vi "OCV Host Client.vi"() -> ()   [LabVIEW 2019]
uses:
  OCVResults.ctl
  <vilib>/NI/STM/TCP/Read Meta Data (TCP Ref).vi
  <vilib>/NI/STM/TCP/Get Connection Reference (TCP).vi
  <vilib>/NI/STM/TCP/Read Meta Data (TCP Clst).vi
  <vilib>/NI/STM/TCP/Write Message (TCP).vi
  <vilib>/NI/STM/TCP/Read Message (TCP).vi
  <vilib>/NI/STM/NI STM.lvlib
panel:
  out "Results":T1={"V ch0 Array"=[-3.6706721797527737e-06, -3.7498129566879645e-06, -4.506527481324882e-06, -3.950514239764907e-06, -3.163693240167565e-06, -4.344248671038362e-06, -4.095274961024307e-06, -3.5751580182405744e-06, -3.679018613642735e-06, -4.241224075624106e-06, -3.987139173161142e-06, -4.095162898018893e-06, -3.847206102337771e-06, -3.5638421272775453e-06, -4.562072176859353e-06, -4.7605988032426154e-06, -4.427579247767526e-06, -3.852601385134958e-06, -4.1020189664170556e-06, -4.3281080989855496e-06, -5.440516492777152e-06, -3.984546752057509e-06, -5.212236089778075e-06, -5.036428159001794e-06, -5.147592315385633e-06, -5.639821151819425e-06, -5.515877149224325e-06, -4.719119249712352e-06, -4.963946714892732e-06, -5.484948605605908e-06, -4.699117481856034e-06, -4.371411013381793e-06], "V ch1 Array"=[3.16348946577608e-07, -4.6006644164974094e-08, 1.3969711256247924e-07, 5.504038021469118e-07, 6.043373546159048e-07, 8.588910763946214e-07, 3.873000478455866e-07, -9.425550832049107e-08, 5.478098926620833e-07, -1.5101867437911976e-08, 5.338250456123853e-07, 2.1443809689103476e-07, 4.7544765511864677e-07, 2.3162631910812704e-07, 8.243432281255722e-07, 4.471382249715257e-08, 5.99790680569682e-08, -2.2315078204485062e-07, 2.9341057780098417e-07, 5.004289692054384e-07, -7.392261536330597e-07, -5.620196062138411e-07, -3.660452758084688e-07, -9.194345360493777e-07, -9.111679257871997e-07, -7.512468979028726e-07, -1.0558354724851492e-06, -7.932704939374199e-07, -5.322755445721049e-07, -1.1027151194362871e-06, -8.832653614145757e-07, -1.2875743851160654e-08], "V ch2 Array"=[9.302674524081596e-06, 9.024588901172551e-06, 9.175881665259862e-06, 9.276460385887776e-06, 8.94756426004191e-06, 9.124853023363049e-06, 8.424398713182681e-06, 8.62613322878038e-06, 8.99729374546172e-06, 9.302350488450816e-06, 9.314432037131127e-06, 9.207132923863602e-06, 8.920051579064495e-06, 8.702882444652302e-06, 9.103302590152476e-06, 8.938969157386832e-06, 8.921195968554336e-06, 8.792009492927474e-06, 9.494545679269322e-06, 9.110247967355348e-06, 8.668435221623828e-06, 7.95156633600334e-06, 8.401197094566e-06, 8.499396743148332e-06, 8.067369388963132e-06, 8.816372879417737e-06, 7.610167561411513e-06, 7.594234882129245e-06, 8.485125121852154e-06, 8.105819415375889e-06, 8.729915422429432e-06, 7.897303713033343e-06], "V ch3 Array"=[7.69393857109199e-06, 8.057167587189197e-06, 7.1228622148927485e-06, 7.424852427233159e-06, 6.8217649437894305e-06, 7.201445944926346e-06, 7.710957721782108e-06, 7.736723821001707e-06, 7.68957282130428e-06, 7.319043173912174e-06, 7.476899876041569e-06, 7.1550863314873234e-06, 7.295375552383249e-06, 7.1219749115015865e-06, 7.996068874298418e-06, 7.215675170715944e-06, 7.2928039847892635e-06, 7.091536693290006e-06, 7.2765313907074405e-06, 7.659634434212023e-06, 7.289115911683562e-06, 6.62300445032373e-06, 6.310563673677977e-06, 6.475814441935722e-06, 6.9014245158358485e-06, 6.608592632669611e-06, 6.07353098569707e-06, 6.0353281126732675e-06, 6.4467487474758576e-06, 6.896290120465679e-06, 7.301165398420061e-06, 6.570120591901739e-06], "V ch4 Array"=[], "Elapsed Time (ms)"=5101, "DMM Fault Array"=[FALSE, FALSE, FALSE, FALSE, FALSE, FALSE, FALSE, FALSE, FALSE, FALSE, FALSE, FALSE, FALSE, FALSE, FALSE, FALSE, FALSE, FALSE, FALSE, FALSE, FALSE, FALSE, FALSE, FALSE, FALSE, FALSE, FALSE, FALSE, FALSE, FALSE, FALSE, FALSE, FALSE, FALSE, FALSE, FALSE, FALSE, FALSE, FALSE, FALSE, FALSE, FALSE, FALSE, FALSE, FALSE, FALSE, FALSE, FALSE, FALSE, FALSE, FALSE, FALSE, FALSE, FALSE, FALSE, FALSE, FALSE, FALSE, FALSE, FALSE, FALSE, FALSE, FALSE, FALSE, FALSE, FALSE, FALSE, FALSE, FALSE, FALSE, FALSE, FALSE, FALSE, FALSE, FALSE, FALSE, FALSE, FALSE, FALSE, FALSE, FALSE, FALSE, FALSE, FALSE, FALSE, FALSE, FALSE, FALSE, FALSE, FALSE, FALSE, FALSE, FALSE, FALSE, FALSE, FALSE, FALSE, FALSE, FALSE, FALSE, FALSE, FALSE, FALSE, FALSE, FALSE, FALSE, FALSE, FALSE, FALSE, FALSE, FALSE, FALSE, FALSE, FALSE, FALSE, FALSE, FALSE, FALSE, FALSE, FALSE, FALSE, FALSE, FALSE, FALSE, FALSE, FALSE, FALSE, FALSE]}
  out "Waveform Graph ch3":dbl[](graph)=[7.69393857109199e-06, 8.057167587189197e-06, 7.1228622148927485e-06, 7.424852427233159e-06, 6.8217649437894305e-06, 7.201445944926346e-06, 7.710957721782108e-06, 7.736723821001707e-06, 7.68957282130428e-06, 7.319043173912174e-06, 7.476899876041569e-06, 7.1550863314873234e-06, 7.295375552383249e-06, 7.1219749115015865e-06, 7.996068874298418e-06, 7.215675170715944e-06, 7.2928039847892635e-06, 7.091536693290006e-06, 7.2765313907074405e-06, 7.659634434212023e-06, 7.289115911683562e-06, 6.62300445032373e-06, 6.310563673677977e-06, 6.475814441935722e-06, 6.9014245158358485e-06, 6.608592632669611e-06, 6.07353098569707e-06, 6.0353281126732675e-06, 6.4467487474758576e-06, 6.896290120465679e-06, 7.301165398420061e-06, 6.570120591901739e-06]
  out "Waveform Graph ch2":dbl[](graph)=[9.302674524081596e-06, 9.024588901172551e-06, 9.175881665259862e-06, 9.276460385887776e-06, 8.94756426004191e-06, 9.124853023363049e-06, 8.424398713182681e-06, 8.62613322878038e-06, 8.99729374546172e-06, 9.302350488450816e-06, 9.314432037131127e-06, 9.207132923863602e-06, 8.920051579064495e-06, 8.702882444652302e-06, 9.103302590152476e-06, 8.938969157386832e-06, 8.921195968554336e-06, 8.792009492927474e-06, 9.494545679269322e-06, 9.110247967355348e-06, 8.668435221623828e-06, 7.95156633600334e-06, 8.401197094566e-06, 8.499396743148332e-06, 8.067369388963132e-06, 8.816372879417737e-06, 7.610167561411513e-06, 7.594234882129245e-06, 8.485125121852154e-06, 8.105819415375889e-06, 8.729915422429432e-06, 7.897303713033343e-06]
  out "Waveform Graph ch1":dbl[](graph)=[3.16348946577608e-07, -4.6006644164974094e-08, 1.3969711256247924e-07, 5.504038021469118e-07, 6.043373546159048e-07, 8.588910763946214e-07, 3.873000478455866e-07, -9.425550832049107e-08, 5.478098926620833e-07, -1.5101867437911976e-08, 5.338250456123853e-07, 2.1443809689103476e-07, 4.7544765511864677e-07, 2.3162631910812704e-07, 8.243432281255722e-07, 4.471382249715257e-08, 5.99790680569682e-08, -2.2315078204485062e-07, 2.9341057780098417e-07, 5.004289692054384e-07, -7.392261536330597e-07, -5.620196062138411e-07, -3.660452758084688e-07, -9.194345360493777e-07, -9.111679257871997e-07, -7.512468979028726e-07, -1.0558354724851492e-06, -7.932704939374199e-07, -5.322755445721049e-07, -1.1027151194362871e-06, -8.832653614145757e-07, -1.2875743851160654e-08]
  out "Scanning":bool
  out "Waveform Graph ch0":dbl[](graph)=[-3.6706721797527737e-06, -3.7498129566879645e-06, -4.506527481324882e-06, -3.950514239764907e-06, -3.163693240167565e-06, -4.344248671038362e-06, -4.095274961024307e-06, -3.5751580182405744e-06, -3.679018613642735e-06, -4.241224075624106e-06, -3.987139173161142e-06, -4.095162898018893e-06, -3.847206102337771e-06, -3.5638421272775453e-06, -4.562072176859353e-06, -4.7605988032426154e-06, -4.427579247767526e-06, -3.852601385134958e-06, -4.1020189664170556e-06, -4.3281080989855496e-06, -5.440516492777152e-06, -3.984546752057509e-06, -5.212236089778075e-06, -5.036428159001794e-06, -5.147592315385633e-06, -5.639821151819425e-06, -5.515877149224325e-06, -4.719119249712352e-06, -4.963946714892732e-06, -5.484948605605908e-06, -4.699117481856034e-06, -4.371411013381793e-06]
  in  "Command":string(combo)="Stop Client"
  out "Error Out":errorcluster={"status"=FALSE, "code"=66, "source"="TCP Read in NI STM.lvlib:Read Message (TCP).vi:6180001->OCV Host Client.vi"}
  in  "Send_Command":bool
  in  "Target IP Address":string="169.254.139.159"
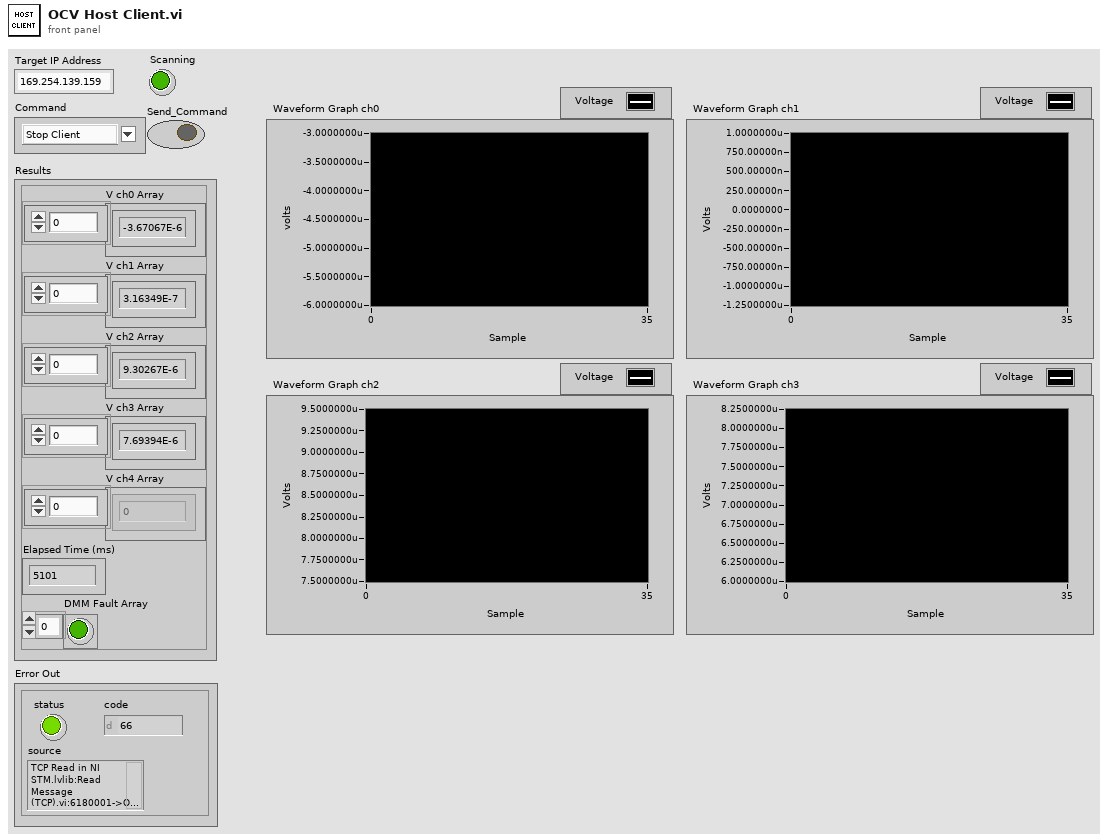
[diagram p1: front panel]
types:
  T1 = typedef "OCVResults.ctl" = cluster{"V ch0 Array":dbl[], "V ch1 Array":dbl[], "V ch2 Array":dbl[], "V ch3 Array":dbl[], "V ch4 Array":dbl[], "Elapsed Time (ms)":u32, "DMM Fault Array":bool[]}
  T2 = typedef "NI STM.lvlib/TCP Connection Info.ctl" = cluster{"connection ID":refnum<k5>, "meta data":T3[]}
  T3 = typedef "NI STM.lvlib/MetaDataElement.ctl" = string
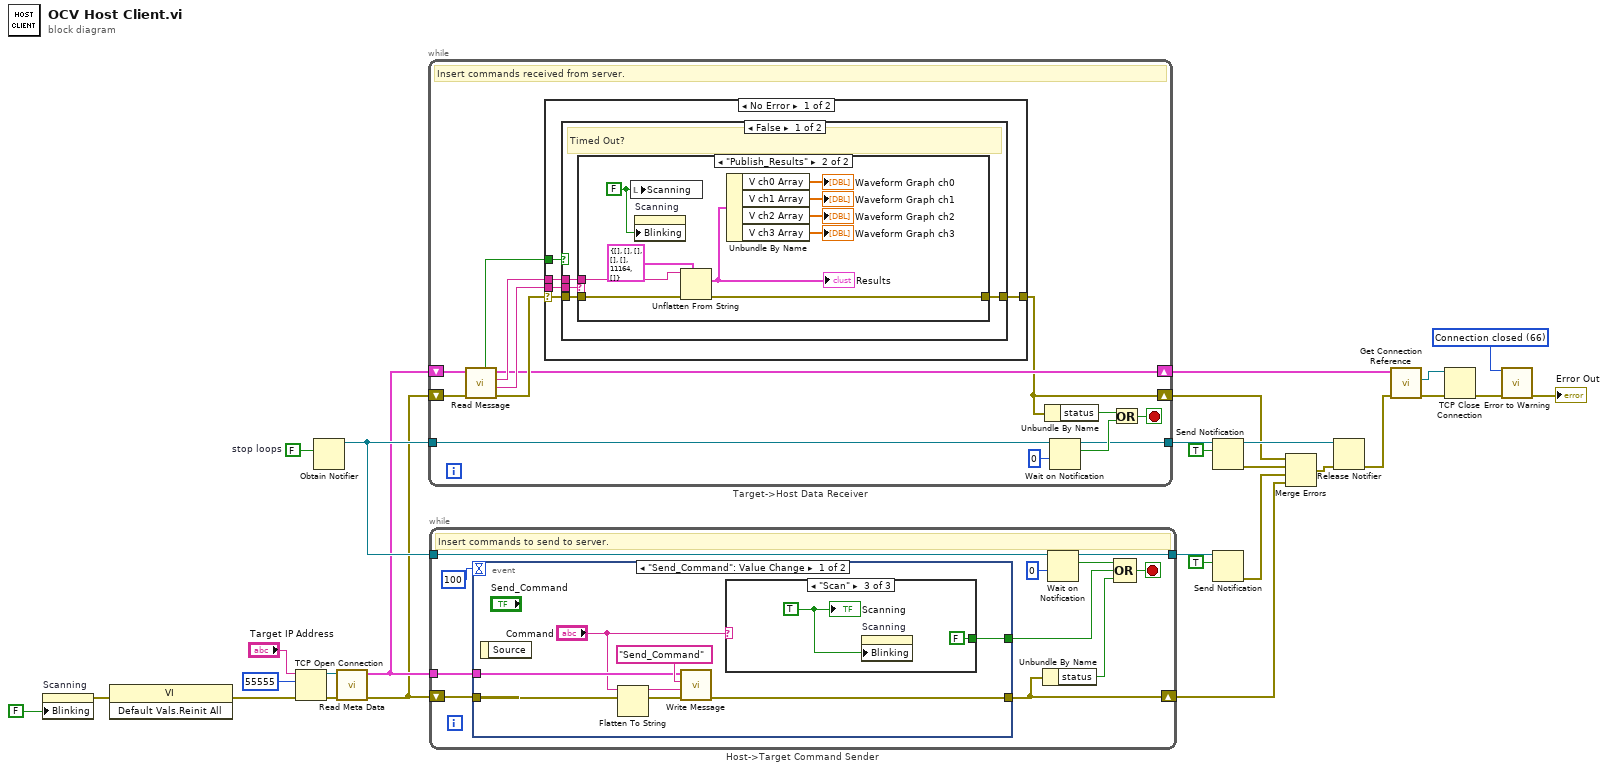
[diagram p0: block diagram]
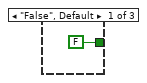
[diagram p2: hidden frame]
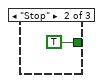
[diagram p3: hidden frame]
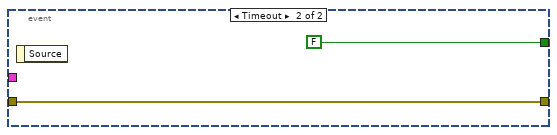
[diagram p4: hidden frame]
diagram:
  w14 = FALSE  # stop loops
  w26 = 66 items=["No Error", "Argument Error", "Memory Full", "Out of Zone", "End of File", "File Already Open", "Generic File IO Error", "File Not Found", "File Permission Error", "Disk Full", "Duplicate Path", "Too Many Files Open", "Not Enabled", "Resource File Not Found", "Cannot Add Resource", "Resource Not Found", "Image Not Found", "Image Memory Error", "Pen Does Not Exist", "Config Bad Type", "Config Token Not Found", "Config Parse Error", "Config Memory Error", "Bad External Code Format", "Bad External Code Offset", "External Code Not Present", "Null Window", "Destroy Window Mixup", "Null Menu", "Print Aborted", "Bad Print Record", "Print Driver Error", "Windows Error During Print", "Memory Error During Print", "Print Dialog Error", "Generic Print Error", "Invalid Device Refnum", "Device Not Found", "Device Parameter Error", "Device Unit Error", "Can't Open Device", "Device Call Aborted", "Generic Error", "Cancelled By User", "Object ID Too Low", "Object ID Too High", "Object Not In Heap", "Unknown Heap", "Bad DefProc ID", "DefProc Not In Table", "Message Out Of Range", "Null Method", "Unknown Message", "Manager Call Not Supported", "Bad address", "Connection In progress", "Connection timed out", "Connection is already in progress", "Network attribute not supported", "Network error", "Address in use", "System out of memory", "Connection aborted", "Connection refused", "Connection is not connected", "Connection is already connected", "Connection closed", "Initialize error (interapplication manager)", "Bad occurrence", "Wait on unbound occurrence handler", "Occurrence queue overflow", "Bad path", "Semaphore not signaled", "Unrecognized type (interapplication manager)"] ("1st Error to Convert")
  n1 = property on="Scanning" class="Bool (strict)"("Blinking"=FALSE ("Scanning")) -> (error out=w1:errorcluster)  [unwired: 2 in, 1 out]
  n2 = invoke class="VI" method="Default Vals.Reinit All"(error in=w1) -> (error out=w3:errorcluster)  [unwired: 2 in, 2 out]
  n3 = TCP Open Connection(address="Target IP Address", remote port or service name=u16 55555 ("remote port"), error in (no error)=w3) -> (connection ID=w10:refnum<k5>, error out=w9:errorcluster)  [unwired: 2 out]
  n4 = Obtain Notifier(notification data type=w14) -> (notifier out=w17:refnum<notifier>)  [unwired: 3 in, 2 out]
  n5 = call-poly <vilib>:"Read Meta Data.vi"("error in"=w9, "connection ID"=w10) -> ("error out"=w11:errorcluster, "connection info out"=w12:T2)  [unwired: 1 in, 7 out]
  n6 = while "Target->Host Data Receiver" {
    shift-right: [w29] -> w6
    shift-left: w11 -> [w41]
    tunnel: w17 -> [w35]
    tunnel: [w31] -> w15
    shift-right: [w36] -> w13
    shift-left: w12 -> [w42]
    stop <- w32 stop-if-true
    # "Insert commands received from server."
    n7 = call-poly <vilib>:"Read Message.vi"("error in"=w41, "connection info in"=w42) -> ("error out"=w37:errorcluster, "name"=w40:T3, "data string"=w39:string, "connection info out"=w36:T2, "timed out?"=w38:bool)  [unwired: 3 in, 2 out]
    n8 = case shown="No Error" w37 {
      selector: w37 -> [w44 w64]
      tunnel: w40 -> [w47 _]
      tunnel: w39 -> [w46 _]
      tunnel: w38 -> [w45 _]
      tunnel: [w43 w64] -> w29
      frame No Error {
        n9 = case shown="False" w45 {
          tunnel: w47 -> [w48 _]
          tunnel: w46 -> [w51 _]
          tunnel: w44 -> [w50 w63]
          tunnel: [w49 w63] -> w43
          frame False {
            # "Timed Out?"
            n10 = case shown="\"Publish_Results\"" w48 {
              tunnel: w51 -> [_ w61]
              tunnel: w50 -> [w52 w62]
              tunnel: [w52 w60] -> w49
              frame Default {
              }
              frame "Publish_Results" {
                w57 = FALSE ("Scanning")
                n11 = local write "Scanning"(w57) -> ()
                n12 = property on="Scanning" class="Bool (strict)"("Blinking"=w57) -> ()  [unwired: 2 in, 2 out]
                n13 = Unflatten From String(type=T1 {"V ch0 Array"=[], "V ch1 Array"=[], "V ch2 Array"=[], "V ch3 Array"=[], "V ch4 Array"=[], "Elapsed Time (ms)"=11164, "DMM Fault Array"=[]} ("Results 2"), binary string=w61, error in (no error)=w62) -> (value=w53:T1, error out=w60:errorcluster)  [unwired: 1 in, 2 out]
                "Results" <- w53
                n14 = Unbundle By Name(w53) -> ("V ch0 Array"=→"Waveform Graph ch0":dbl[], "V ch1 Array"=→"Waveform Graph ch1":dbl[], "V ch2 Array"=→"Waveform Graph ch2":dbl[], "V ch3 Array"=→"Waveform Graph ch3":dbl[])
              }
            }
          }
          frame True {
            # "Timed Out?"
          }
        }
      }
      frame Error {
      }
    }
    n15 = Unbundle By Name(w29) -> ("status"=w30:bool)
    n16 = Wait on Notification(notifier=w35, timeout in ms (-1)=0) -> (notifier out=w31:refnum<notifier>, notification=w33:bool)  [unwired: 2 in, 2 out]
    n17 = Or(x=w30, y=w33) -> (x .or. y?=w32:bool)
  }
  n18 = while "Host->Target Command Sender" {
    shift-right: [w67] -> w20
    shift-left: w11 -> [w75]
    tunnel: w12 -> [w74]
    tunnel: w17 -> [w71]
    tunnel: [w68] -> w18
    stop <- w69 stop-if-true
    # "Insert commands to send to server."
    n19 = event shown="[0] \"Send_Command\": Value Change" {
      selector: _ -> [_ _]
      dyn-events: _ -> [_ _]
      timeout: 100 -> [_ _]
      tunnel: w74 -> [w81 _]
      tunnel: w75 -> [w80 w88]
      tunnel: [w76 FALSE ("stop")] -> w66
      tunnel: [w78 w88] -> w67
      event "Send_Command": Value Change {
        n20 = event-data() -> ()  [unwired: 2 out]
        n21 = Flatten To String(anything="Command") -> (data string=w79:string)  [unwired: 2 in, 3 out]
        n22 = call-poly <vilib>:"Write Message.vi"("error in"=w80, "data"=w79, "name"="Send_Command" ("Name"), "connection info in"=w81) -> ("error out"=w78:errorcluster)  [unwired: 1 in, 6 out]
        n23 = case shown="\"Scan\"" "Command" {
          tunnel: [FALSE ("stop") TRUE ("stop") FALSE ("stop")] -> w76
          frame "False", Default {
          }
          frame "Stop" {
          }
          frame "Scan" {
            w85 = TRUE ("Scanning")
            n24 = property on="Scanning" class="Bool (strict)"("Blinking"=w85) -> ()  [unwired: 2 in, 2 out]
            "Scanning" <- w85
          }
        }
      }
      event Timeout {
        n25 = event-data() -> ()  [unwired: 2 out]
      }
    }
    n26 = Unbundle By Name(w67) -> ("status"=w65:bool)
    n27 = Wait on Notification(notifier=w71, timeout in ms (-1)=0) -> (notifier out=w68:refnum<notifier>, notification=w73:bool)  [unwired: 2 in, 2 out]
    n28 = Compound Arithmetic op=OR(w73, w66, w65) -> (w69:bool)
  }
  n29 = Send Notification(notification=TRUE, notifier=w15) -> (notifier out=w23:refnum<notifier>, error out=w22:errorcluster)  [unwired: 1 in]
  n30 = Send Notification(notification=TRUE, notifier=w18) -> (error out=w21:errorcluster)  [unwired: 1 in, 1 out]
  n31 = Merge Errors(w6, w22, w21, w20) -> (w24:errorcluster)
  n32 = Release Notifier(notifier=w23, error in (no error)=w24) -> (error out=w25:errorcluster)  [unwired: 1 in, 2 out]
  n33 = call-poly <vilib>:"Get Connection Reference.vi"("error in"=w25, "connection info in"=w13) -> ("error out"=w5:errorcluster, "connection ID out"=w4:refnum<k5>)  [unwired: 8 out]
  n34 = TCP Close Connection(connection ID=w4, error in (no error)=w5) -> (error out=w27:errorcluster)  [unwired: 2 out]
  n35 = call <vilib>:"Error to Warning.vi"("1st Error to Convert"=w26, "error in"=w27) -> ("warning out"=→"Error Out":errorcluster)  [unwired: 3 in, 10 out]
